vi "Convert Test Status To Colourbox.vi"(11 "Test Result":T2) -> (3 "Status":T1)   [LabVIEW 2015]
uses:
  Application Specific/Drivers/PLC Modbus/Test Status.ctl
  Application Specific/Controls/Test Status Colourbox (Large).ctl
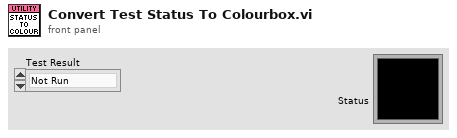
[diagram p1: front panel]
types:
  T1 = typedef "Utility.lvlib/Test Status Colourbox (Large).ctl" = u32
  T2 = typedef "Utility.lvlib/Test Status.ctl" = enum32{"Not Run", "In Progress", "Pass", "Fail", "N/A"}
  T3 = typedef "Constants.ctl" = cluster{"Colours":cluster{"OK":u32, "Warning":u32, "Error":u32, "Green On":u32, "Green Off":u32, "Red On":u32, "Red Off":u32}, "System":cluster{"Target Frames Second":dbl, "Field Size":T4, "Window Size":T4, "Viewport Size":T4, "Sidebar Scaling":sgl, "Sidebar Width":i32}, "Game":cluster{"Maximum Asteroids":i32, "Max Energy":i32, "Max Crew":i32}}
  T4 = typedef "Math.lvlib/Point (I32).ctl" = cluster{"x":i32, "y":i32}
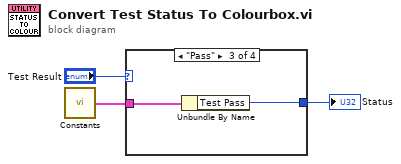
[diagram p0: block diagram]
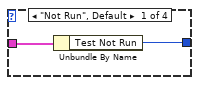
[diagram p2: hidden frame]
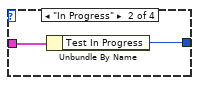
[diagram p3: hidden frame]
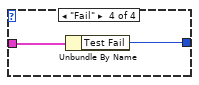
[diagram p4: hidden frame]
diagram:
  n1 = call "Constants.vi"() -> ("Constants"=w2:T3)
  n2 = case shown="\"Pass\"" "Test Result" {
    tunnel: w2 -> [w5 w7 w9 w11]
    tunnel: [w4 w6 w8 w10] -> w1
    frame "Not Run", Default {
      n3 = Unbundle By Name(w5) -> ("Test Not Run"=w4:u32)
    }
    frame "In Progress" {
      n4 = Unbundle By Name(w7) -> ("Test In Progress"=w6:u32)
    }
    frame "Pass" {
      n5 = Unbundle By Name(w9) -> ("Test Pass"=w8:u32)
    }
    frame "Fail" {
      n6 = Unbundle By Name(w11) -> ("Test Fail"=w10:u32)
    }
  }
  "Status" <- w1
